vi "Create (Group).vi"(8 "error in (no error)":errorcluster, 10 "Group Config":refnum<class "Group.lvclass">) -> (0 "error out":errorcluster, 3 "VolatusScaling out":refnum<class "Scaling.lvclass">)   [LabVIEW 2020, in "VolatusData.lvlib" / "Scaling.lvclass"]
uses:
  Scaling.lvclass
  Scaling.lvclass/Scaling.ctl
  VolatusConfig/Scaling/Scaling.lvclass
  VolatusConfig/Group/Group.lvclass
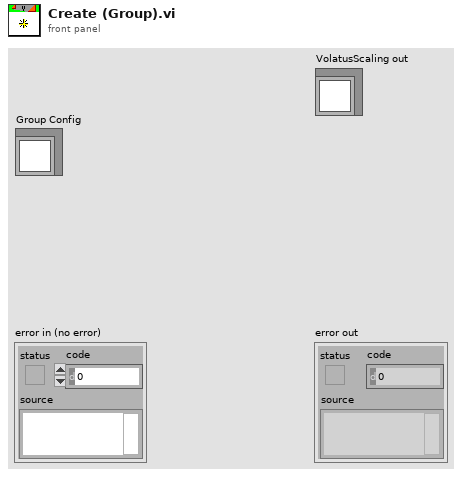
[diagram p1: front panel]
types:
  T1 = typedef "VolatusConfig.lvlib/Scale Type.ctl" = enum16{"None", "Sensor", "Polynomial", "Threshold", "Invert Bool"}
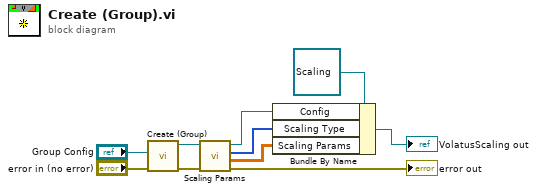
[diagram p0: block diagram]
diagram:
  n1 = call "Create (Group).vi"("error in (no error)"="error in (no error)", "Group Config"="Group Config") -> ("error out"=w5:errorcluster, "Scaling out"=w6:refnum<class "Scaling.lvclass">)  [unwired: 8 in]
  n2 = call "Scaling Params.vi"("error in (no error)"=w5, "Scaling in"=w6) -> ("error out"=→"error out":errorcluster, "Scale Params"=w3:dbl[][], "Scale Types"=w2:T1[], "Scaling out"=w1:refnum<class "Scaling.lvclass">)  [unwired: 6 in]
  n3 = Bundle By Name(cluster=refnum<class "Scaling.lvclass"> refnum ("VolatusScaling in"), "Config"=w1, "Scaling Type"=w2, "Scaling Params"=w3) -> (→"VolatusScaling out":refnum<class "Scaling.lvclass">)
